vi "meTEC_Check for Communication Error.vi"(8 "error in (no error)":errorcluster, 11 "Serial Message_IN":string) -> (0 "error out":errorcluster, 3 "Serial Message_OUT":string)   [LabVIEW 2019]
panel:
  # "--- Outputs ---"
  # "--- Inputs ---"
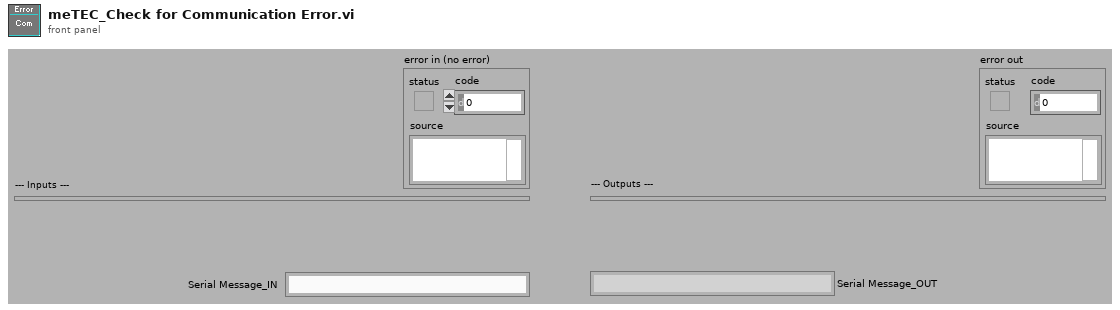
[diagram p1: front panel]
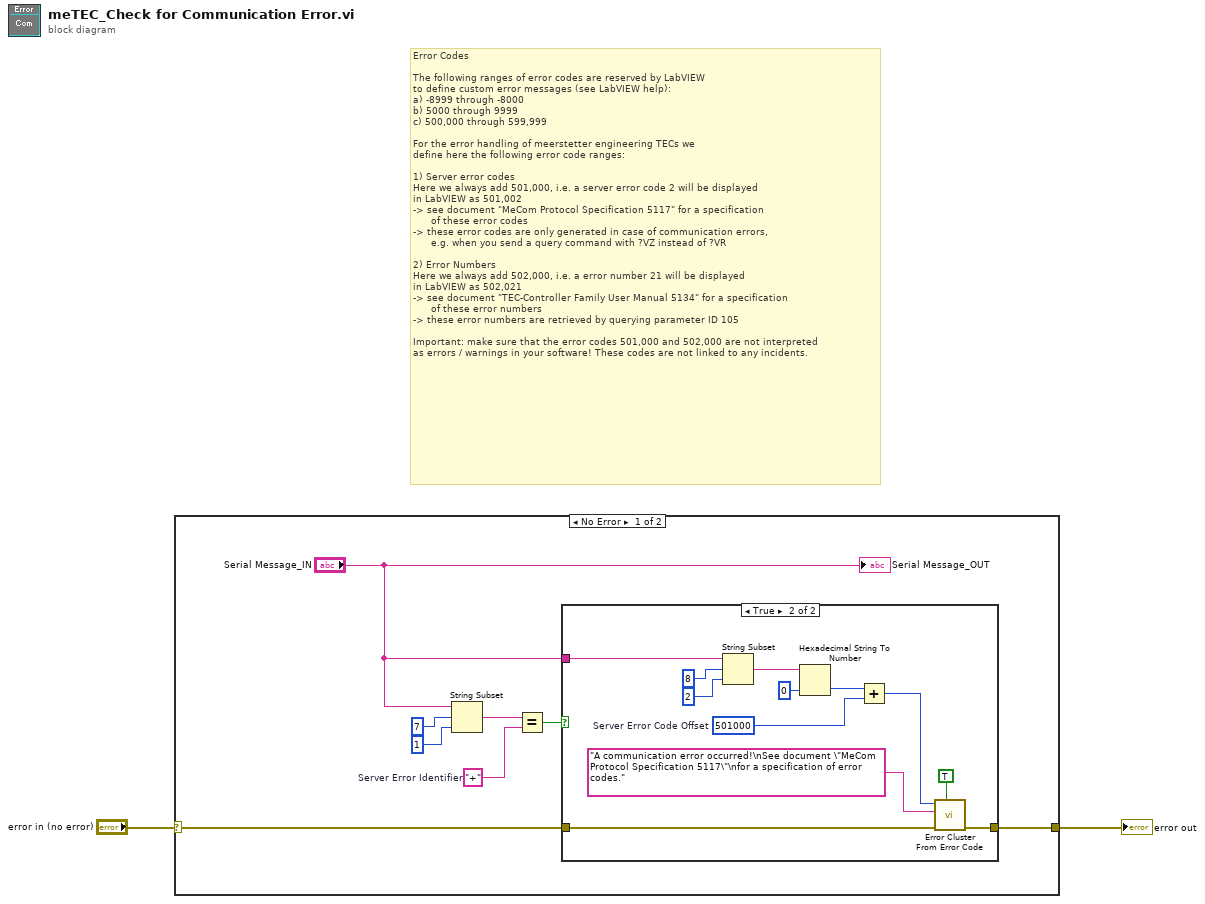
[diagram p0: block diagram]
diagram:
  # "Error Codes\n\nThe following ranges of error codes are reserved by LabVIEW\nto define custom error messages (see LabVIEW help):\na) -8999 through -8000 \nb) 5000 through 9999 \nc) 500,000 through 599,999\n\nFor the error handling of meerstetter engineering TECs we\ndefine here the following error code ranges:\n\n1) Server error codes\nHere we always add 501,000, i.e. a server error code 2 will be displayed\nin LabVIEW as 501,002\n-> see document \"MeCom Protocol Specification 5117\" for a specification \n      of these error codes\n-> these error codes are only generated in case of communication errors, \n      e.g. when you send a query command with ?VZ instead of ?VR \n\n2) Error Numbers\nHere we always add 502,000, i.e. a error number 21 will be displayed\nin LabVIEW as 502,021 \n-> see document \"TEC-Controller Family User Manual 5134\" for a specification \n      of these error numbers\n-> these error numbers are retrieved by querying parameter ID 105 \n\nImportant: make sure that the error codes 501,000 and 502,000 are not interpreted\nas errors / warnings in your software! These codes are not linked to any incidents."
  n1 = case shown="No Error" "error in (no error)" {
    selector: "error in (no error)" -> [w4 w24]
    tunnel: [w3 w24] -> w2
    frame No Error {
      w7 = "+"  # Server Error Identifier
      n2 = String Subset(string="Serial Message_IN", offset (0)=7, length (rest)=1 ("length (rest)")) -> (substring=w8:string)
      n3 = Equal?(x=w8, y=w7) -> (x = y?=w6:bool)
      n4 = case shown="True" w6 {
        tunnel: "Serial Message_IN" -> [_ w21]
        tunnel: [w11 w15] -> w3
        tunnel: w4 -> [w11 w12]
        frame False {
        }
        frame True {
          w13 = 501000  # Server Error Code Offset
          n5 = String Subset(string=w21, offset (0)=8, length (rest)=2 ("length (rest)")) -> (substring=w19:string)
          n6 = Hexadecimal String To Number(string=w19, default (0uL)=0 ("default (0 U32)")) -> (number=w18:i32)  [unwired: 1 in, 1 out]
          n7 = Add(x=w18, y=w13) -> (x+y=w17:i32)
          n8 = call <vilib>:"Error Cluster From Error Code.vi"("show call chain? (False)"=TRUE, "error in (no error)"=w12, "error message (\"\")"="A communication error occurred!\nSee document \"MeCom Protocol Specification 5117\"\nfor a specification of error codes." ("error message (\"\")"), "error code (0)"=w17) -> ("error out"=w15:errorcluster)  [unwired: 5 in]
        }
      }
      "Serial Message_OUT" <- "Serial Message_IN"
    }
    frame Error {
    }
  }
  "error out" <- w2
